vi "Parse_Recipe.vi"(8 "error in (no error)":errorcluster, 9 "Step In":i32, 10 "Recipe":i32, 11 "Recipes":string[][](array[string])=[["1", "Rice", "66PL10", "12PL3", "10PL4"], ["2", "Frozen Dinner", "5PL8", "10PL2", ""], ["3", "Popcorn", "5PL3", "", ""]]) -> (0 "error out":errorcluster, 1 "PL":string, 2 "Food":string, 3 "Time Remaining":dbl, 5 "Number of Steps":i32)   [LabVIEW 2026]
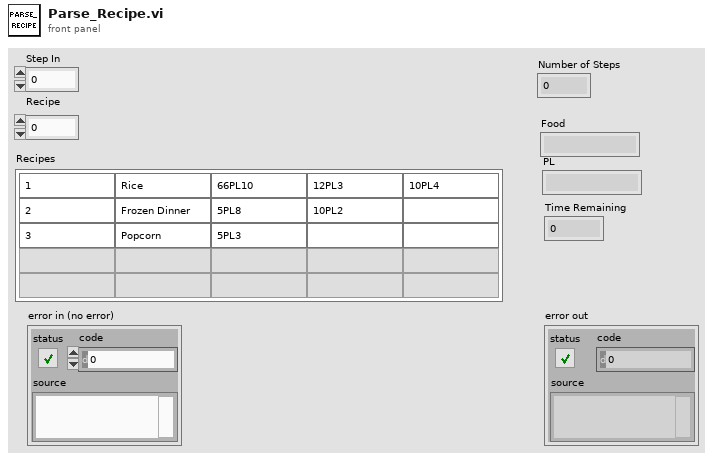
[diagram p1: front panel]
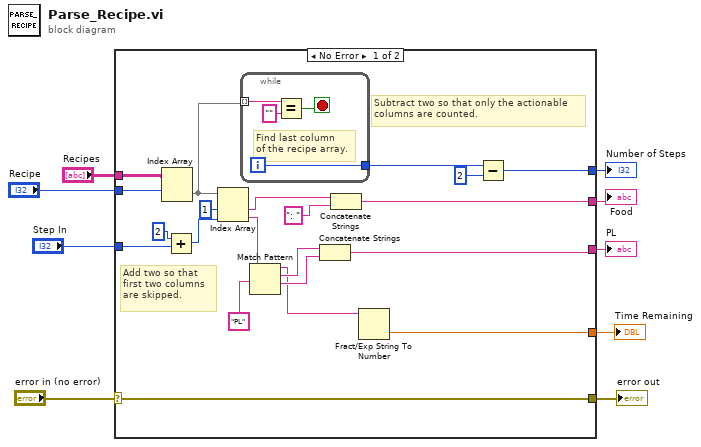
[diagram p0: block diagram]
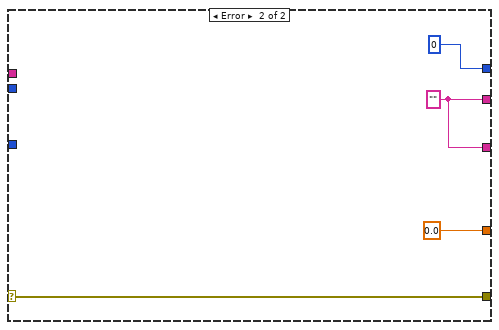
[diagram p2: hidden frame]
diagram:
  n1 = case shown="No Error" "error in (no error)" {
    selector: "error in (no error)" -> [w17 w38]
    tunnel: [w24 0.0] -> w9
    tunnel: "Recipes" -> [w23 _]
    tunnel: "Recipe" -> [w22 _]
    tunnel: "Step In" -> [w21 _]
    tunnel: [w17 w38] -> w4
    tunnel: [w16 w36] -> w2
    tunnel: [w15 w36] -> w3
    tunnel: [w11 0] -> w1
    frame No Error {
      # "Add two so that\nfirst two columns\nare skipped."
      # "Subtract two so that only the actionable\ncolumns are counted."
      n2 = Index Array(array=w23, index (row)=w22) -> (element=w13:string[])  [unwired: 1 in]
      n3 = Add(x=2, y=w21) -> (x+y=w27:i32)
      n4 = Index Array(array=w13, index #1=1 ("index"), index #2=w27) -> (element #1=w20:string, element #2=w19:string)
      n5 = while {
        tunnel: w13 -> [w34] mode=indexing
        tunnel: [w31] -> w12
        i -> [w31]
        stop <- w32 stop-if-true
        # "Find last column\nof the recipe array."
        n6 = Equal?(x=w34, y="") -> (x = y?=w32:bool)
      }
      n7 = Match Pattern(string=w19, regular expression="PL") -> (before substring=w14:string, match substring=w28:string, after substring=w18:string)  [unwired: 1 in, 1 out]
      n8 = Concatenate Strings(w28, w18) -> (w15:string)
      n9 = Concatenate Strings(w20, ": ") -> (w16:string)
      n10 = Fract/Exp String To Number(string=w14) -> (number=w24:dbl)  [unwired: 3 in, 1 out]
      n11 = Subtract(x=w12, y=2) -> (x-y=w11:i32)
    }
    frame Error {
      w36 = ""
    }
  }
  "Time Remaining" <- w9
  "error out" <- w4
  "PL" <- w3
  "Food" <- w2
  "Number of Steps" <- w1
